vi "Joysticks to Drive Motors.vi"(8 "Boost?":bool, 9 "Turn":dbl, 10 "Throttle":dbl) -> (2 "Drive Motor Values":cluster{"Left Motor":dbl, "Right Motor":dbl})   [LabVIEW 2018]
uses:
  Robot Global Data.vi
  Infrastructure/Constants.vi
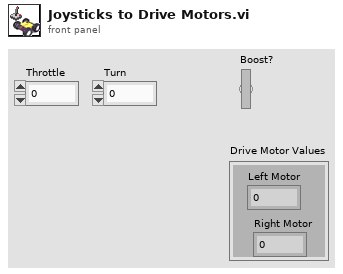
[diagram p1: front panel]
types:
  T1 = cluster{"Left Motor Value":dbl, "Right Motor Value":dbl}
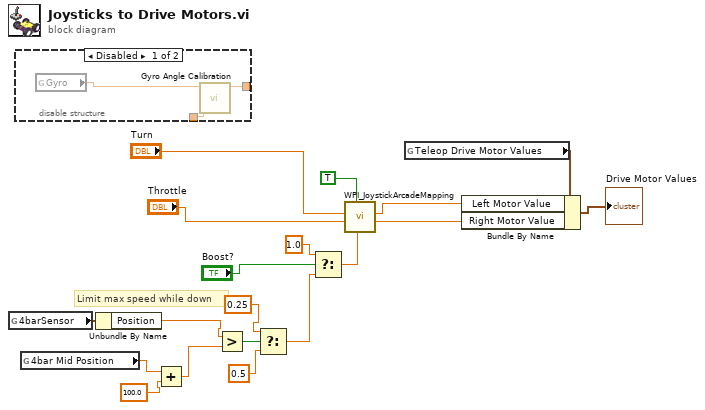
[diagram p0: block diagram]
diagram:
  # "Limit max speed while down"
  n1 = global read "Robot Global Data.vi" "4barSensor"() -> (w9:cluster{"Position":dbl, "Velocity":dbl})
  n2 = disable-structure shown="Disabled" {
    disable-tunnel: _ -> [w22 _]
    disable-tunnel: [w21 _] -> _
    frame Disabled {
      n3 = global read "Robot Global Data.vi" "Gyro"() -> (w20:dbl)
      n4 = call "Gyro Angle Calibration.vi"("turning joystick input"=w22, "Gyro"=w20) -> ("adjusted turning output"=w21:dbl)  [unwired: 9 in]
    }
    frame Enabled {
    }
  }
  n5 = global read "Constants.vi" "4bar Mid Position"() -> (w3:dbl)
  n6 = Unbundle By Name(w9) -> ("Position"=w4:dbl)
  n7 = Add(x=w3, y=100.0) -> (x+y=w2:dbl)
  n8 = Greater?(x=w4, y=w2) -> (0:w5:bool)
  n9 = Select(t=0.25 ("Max Output"), s=w5, f=0.5 ("Max Output")) -> (s? t:f=w6:dbl)
  n10 = Select(t=1.0 ("Max Output"), s="Boost?", f=w6) -> (s? t:f=w19:dbl)
  n11 = call <vilib>:"WPI_JoystickArcadeMapping.vi"("Max Output"=w19, "Square Inputs"=TRUE, "Y axis value"="Throttle", "X axis value"="Turn") -> ("Right Motor Value"=w12:dbl, "Left Motor Value"=w13:dbl)  [unwired: 6 in]
  n12 = global read "Robot Global Data.vi" "Teleop Drive Motor Values"() -> (w14:T1)
  n13 = Bundle By Name(cluster=w14, "Left Motor Value"=w13, "Right Motor Value"=w12) -> (→"Drive Motor Values":T1)
